vi "Create UI.vi"(8 "error in (no error)":errorcluster, 10 "Instrument":refnum<class "Instrument.lvclass">, 11 "Instrument.VoltageSource UI.lvclass":refnum<class "Instrument.VoltageSource UI.lvclass">) -> (0 "error out":errorcluster, 3 "Instrument.VoltageSource UI.lvclass":refnum<class "Instrument.VoltageSource UI.lvclass">)   [LabVIEW 2016, in "Instrument.VoltageSource UI.lvclass"]
uses:
  Instrument.VoltageSource UI.lvclass
  C:/Program Files (x86)/National Instruments/LabVIEW 2016/vi.lib/JKI/JKI SMO/SMO/SMO.lvclass
  <userlib>/LevyLab/Levylab Instruments/SMOs/Instrument/Instrument.lvclass
  Instrument.VoltageSource UI.lvclass/Instrument.VoltageSource UI.ctl
  <vilib>/JKI/JKI SMO/SMO/SMO.lvclass
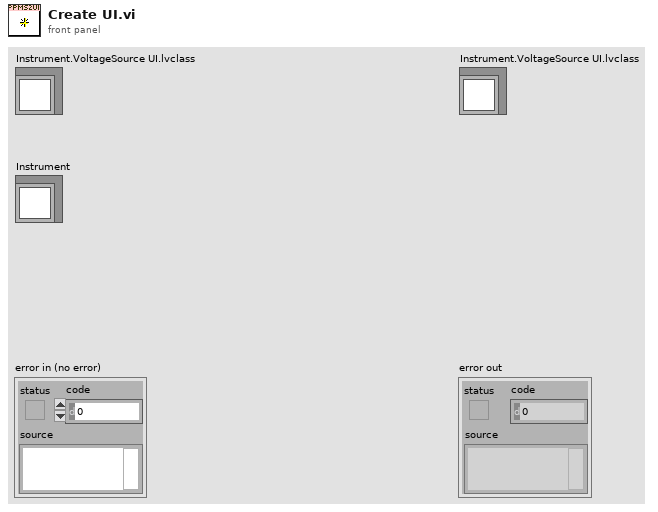
[diagram p1: front panel]
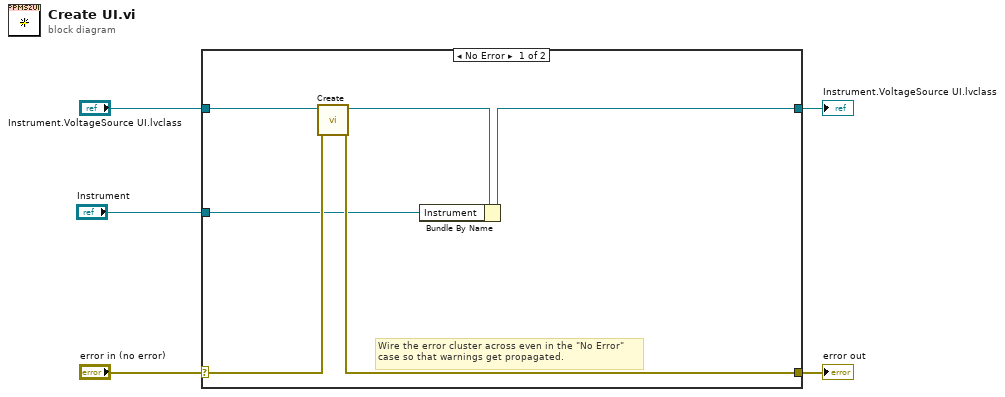
[diagram p0: block diagram]
diagram:
  n1 = case shown="No Error" "error in (no error)" {
    selector: "error in (no error)" -> [w8 w13]
    tunnel: [w7 w13] -> w4
    tunnel: [w11 w12] -> w2
    tunnel: "Instrument.VoltageSource UI.lvclass" -> [w10 w12]
    tunnel: "Instrument" -> [w6 _]
    frame No Error {
      # "Wire the error cluster across even in the \"No Error\"\ncase so that warnings get propagated."
      n2 = call <vilib>:"Create.vi"("error in (no error)"=w8, "SMO"=w10) -> ("error out"=w7:errorcluster, "SMO out"=w9:refnum<class "Instrument.VoltageSource UI.lvclass">)  [unwired: 7 in, 1 out]
      n3 = Bundle By Name(cluster=w9, "Instrument"=w6) -> (w11:refnum<class "Instrument.VoltageSource UI.lvclass">)
    }
    frame Error {
    }
  }
  "error out" <- w4
  "Instrument.VoltageSource UI.lvclass" <- w2
